vi "Waveform data class VI - retrieve total displacement data.vi"(8 "error in (no error)":errorcluster, 11 "Waveform data in":refnum<class "Waveform data.lvclass">) -> (0 "error out":errorcluster, 2 "net total displacement":dbl, 3 "Waveform data out":refnum<class "Waveform data.lvclass">)   [LabVIEW 2010, in "Waveform data.lvclass"]
uses:
  Waveform data.lvclass
  Waveform data.lvclass/Waveform data.ctl
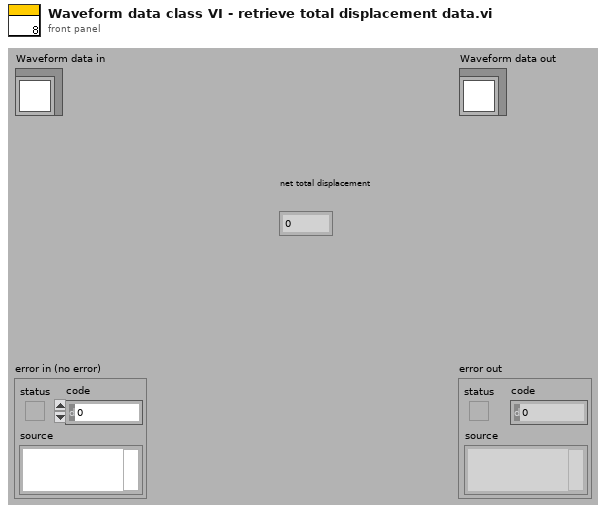
[diagram p1: front panel]
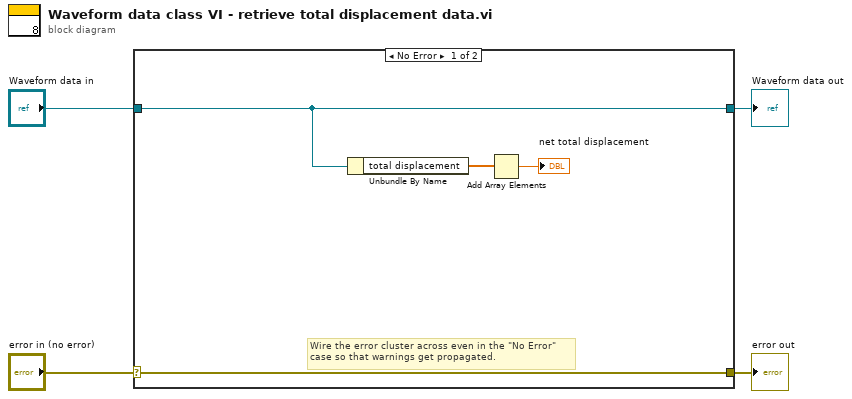
[diagram p0: block diagram]
diagram:
  n1 = case shown="No Error" "error in (no error)" {
    selector: "error in (no error)" -> [w8 w10]
    tunnel: [w8 w10] -> w3
    tunnel: [w7 w9] -> w1
    tunnel: "Waveform data in" -> [w7 w9]
    frame No Error {
      # "Wire the error cluster across even in the \"No Error\"\ncase so that warnings get propagated."
      n2 = Unbundle By Name(w7) -> ("total displacement"=w6:dbl[])
      n3 = Add Array Elements(numeric array=w6) -> (sum=→"net total displacement":dbl)
    }
    frame Error {
    }
  }
  "error out" <- w3
  "Waveform data out" <- w1
